vi "ex_2.vi"() -> ()   [LabVIEW 2020]
panel:
  in  "Number of points":i32=1000
  out "Waveform Graph 2":dbl[][](graph)
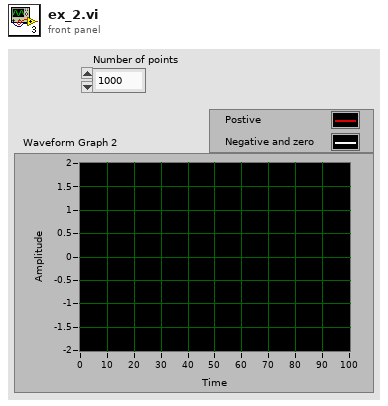
[diagram p1: front panel]
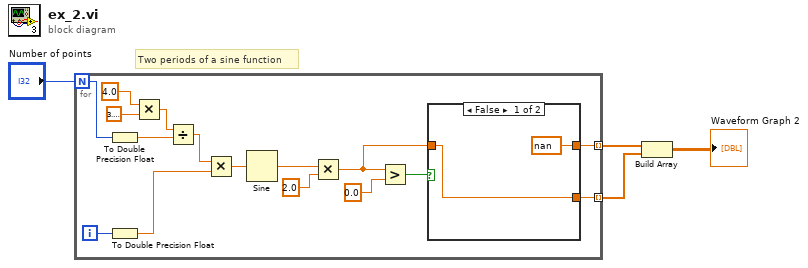
[diagram p0: block diagram]
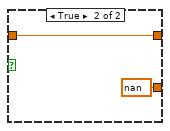
[diagram p2: hidden frame]
diagram:
  # "Two periods of a sine function"
  n1 = for {
    N: "Number of points" -> [w20]
    tunnel: [w6] -> w3 mode=indexing
    tunnel: [w5] -> w2 mode=indexing
    i -> [w18]
    n2 = To Double Precision Float(number=w20) -> (double precision float=w15:dbl)
    n3 = To Double Precision Float(number=w18) -> (double precision float=w17:dbl)
    n4 = Multiply(x=4.0, y=3.141592653589793) -> (x*y=w10:dbl)
    n5 = Divide(x=w10, y=w15) -> (x/y=w19:dbl)
    n6 = Multiply(x=w19, y=w17) -> (x*y=w16:dbl)
    n7 = Sine(x=w16) -> (sin(x)=w14:dbl)
    n8 = Multiply(x=w14, y=2.0) -> (x*y=w7:dbl)
    n9 = Greater?(x=w7, y=0.0) -> (0:w8:bool)
    n10 = case shown="False" w8 {
      tunnel: w7 -> [w22 w24]
      tunnel: [nan w24] -> w6
      tunnel: [w22 nan] -> w5
      frame False {
      }
      frame True {
      }
    }
  }
  n11 = Build Array(w3, w2) -> (→"Waveform Graph 2":dbl[][])
